vi "Build Square Marker Object Points.vi"(1 "Square Length":dbl) -> (0 "Points":T1[](array[typedef]))   [LabVIEW 2020, in "g_ar_toolkit.ar.lvlib"]
uses:
  g_ar_toolkit.ar.lvlib
  g_ar_toolkit.common/Object Point (Float).ctl
  g_ar_toolkit.common/g_ar_toolkit.common.lvlib
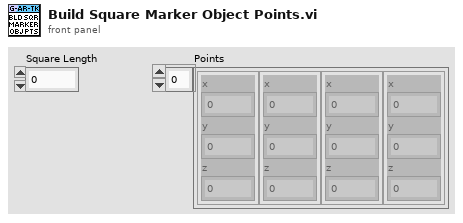
[diagram p1: front panel]
types:
  T1 = typedef "g_ar_toolkit.common.lvlib/Object Point (Float).ctl" = cluster{"x":dbl, "y":dbl, "z":dbl}
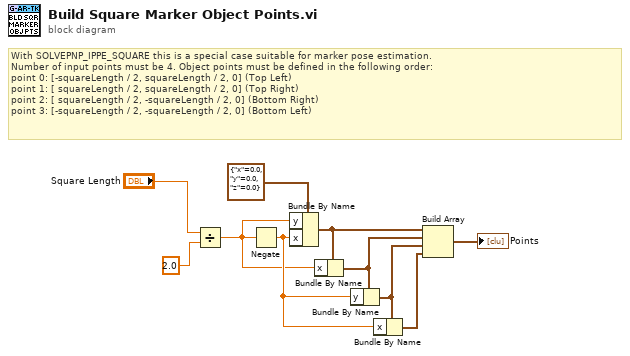
[diagram p0: block diagram]
diagram:
  # "With SOLVEPNP_IPPE_SQUARE this is a special case suitable for marker pose estimation. \nNumber of input points must be 4. Object points must be defined in the following order:\npoint 0: [-squareLength / 2, squareLength / 2, 0] (Top Left)\npoint 1: [ squareLength / 2, squareLength / 2, 0] (Top Right)\npoint 2: [ squareLength / 2, -squareLength / 2, 0] (Bottom Right)\npoint 3: [-squareLength / 2, -squareLength / 2, 0] (Bottom Left)"
  n1 = Divide(x="Square Length", y=2.0) -> (x/y=w5:dbl)
  n2 = Negate(x=w5) -> (-x=w8:dbl)
  n3 = Bundle By Name(cluster=T1 {"x"=0.0, "y"=0.0, "z"=0.0} ("Object Point"), "y"=w5, "x"=w8) -> (w4:T1)
  n4 = Bundle By Name(cluster=w4, "x"=w5) -> (w6:T1)
  n5 = Bundle By Name(cluster=w6, "y"=w8) -> (w7:T1)
  n6 = Bundle By Name(cluster=w7, "x"=w8) -> (w9:T1)
  n7 = Build Array(w4, w6, w7, w9) -> (→"Points":T1[])
